vi "更新动子1&2状态.vi"() -> (0 "Frist ColData":string, 1 "UpDateData":string[](array[string]), 2 "tablename":string, 3 "UpDateCol":string[](array[string]))   [LabVIEW 2017]
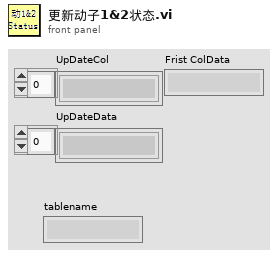
[diagram p1: front panel]
types:
  T1 = typedef "data格式选项.ctl" = enum16{"生成格式", "加载格式"}
  T2 = typedef "缓存操作选项.ctl" = enum16{"初始化", "量测缓存写入", "前侧获取索引", "后侧获取索引", "前侧更新索引", "后侧更新索引", "获取寄存器"}
  T3 = typedef "Data_CT索引操作缓存.ctl" = cluster{"当前data行索引":i32[], "data更新获取索引":T4, "前排提取行号":string, "后排提取行号":string, "当前量测站行号":string, "当前_datetime":string, "量测站操作table缓存":string[], "前排提取_datetime":string, "后排提取_datetime":string}
  T4 = typedef "data更新获取索引.ctl" = cluster{"data更新索引":i32, "前侧获取索引":i32, "后侧获取索引":i32}
  T5 = typedef "表头集合.ctl" = cluster{"product信息":T6, "CT信息":T7, "ER信息":T8, "IOT信息":T9}
  T6 = typedef "product信息.ctl" = cluster{"product表头整合":string[], "量测部分表头":string[], "前侧贴合表头":string[], "后侧贴合表头":string[]}
  T7 = typedef "CT信息.ctl" = cluster{"CT表头整合":string[], "量测CT":string[], "动子1_2CT":string[], "动子3_4CT":string[]}
  T8 = typedef "ER信息.ctl" = cluster{"ER表头整合":string[]}
  T9 = typedef "IOT信息.ctl" = cluster{"IOT表头整合":string[]}
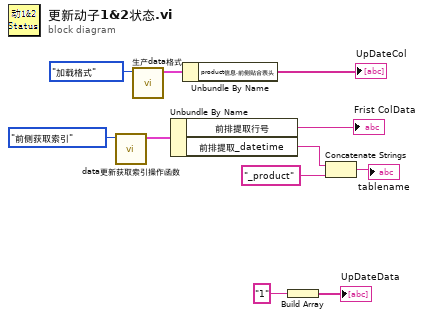
[diagram p0: block diagram]
diagram:
  n1 = call "data更新获取索引操作函数.vi"("缓存操作选项"=缓存操作选项."前侧获取索引") -> ("Data_CT索引操作缓存"=w8:T3)  [unwired: 9 in, 1 out]
  n2 = call "生产data格式.vi"("data格式选项"=data格式选项."加载格式") -> ("表头格式"=w9:T5)  [unwired: 10 in]
  n3 = Unbundle By Name(w8) -> ("前排提取行号"=→"Frist ColData":string, "前排提取_datetime"=w3:string)
  n4 = Unbundle By Name(w9) -> ("product信息.前侧贴合表头"=→"UpDateCol":string[])
  n5 = Build Array("1") -> (→"UpDateData":string[])
  n6 = Concatenate Strings(w3, "_product" ("字符串")) -> (→"tablename":string)
